vi "extract position data.vi"(0 "Receive data":string, 2 "Pre X_M":string, 3 "Pre Y_M":string, 4 "Pre Z_M":string, 5 "Pre X_A":string, 6 "Pre Y_A":string, 7 "Pre Z_A":string) -> (9 "X_A":string, 11 "Y_A":string, 14 "Address":string, 15 "Z_A":string, 16 "Function Code":string, 17 "A_A":string, 20 "X_M":string, 21 "Y_M":string, 23 "Z_M":string, 24 "A_M":string, 27 "CheckSumCorrect":bool)   [LabVIEW 2014, in "HPCNC.lvlib"]
uses:
  HPCNC.lvlib
  GetCncPosition.dll
  mosbusCheckSum.dll
panel:
  in  "dataToGet":i32
  out "length check":string
  out "ChkSumData":u32
  out "AaIdx":u8
  out "ZaIdx":u8
  out "YaIdx":u8
  out "XaIdx":u8
  out "AmIdx":u8
  out "ZmIdx":u8
  out "YmIdx":u8
  out "XmIdx":u8
  out "ChkSumCalculated":u8
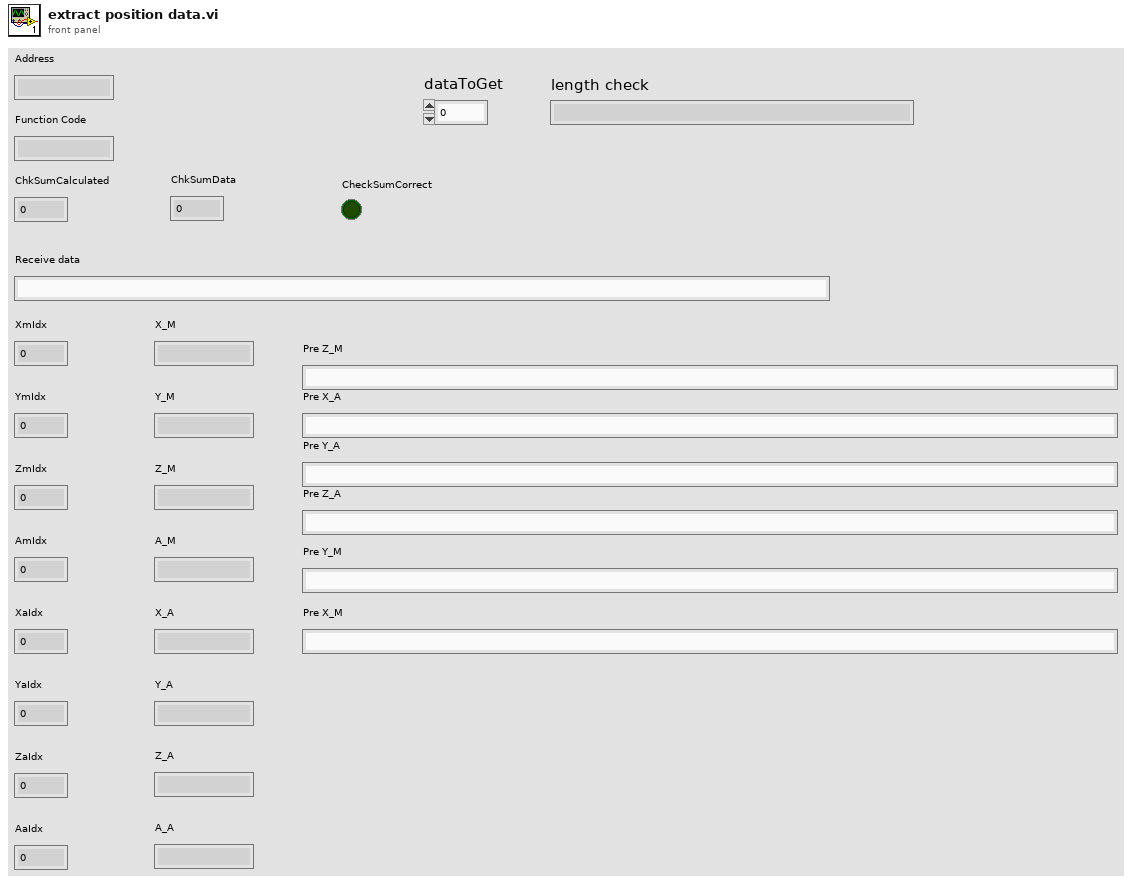
[diagram p1: front panel]
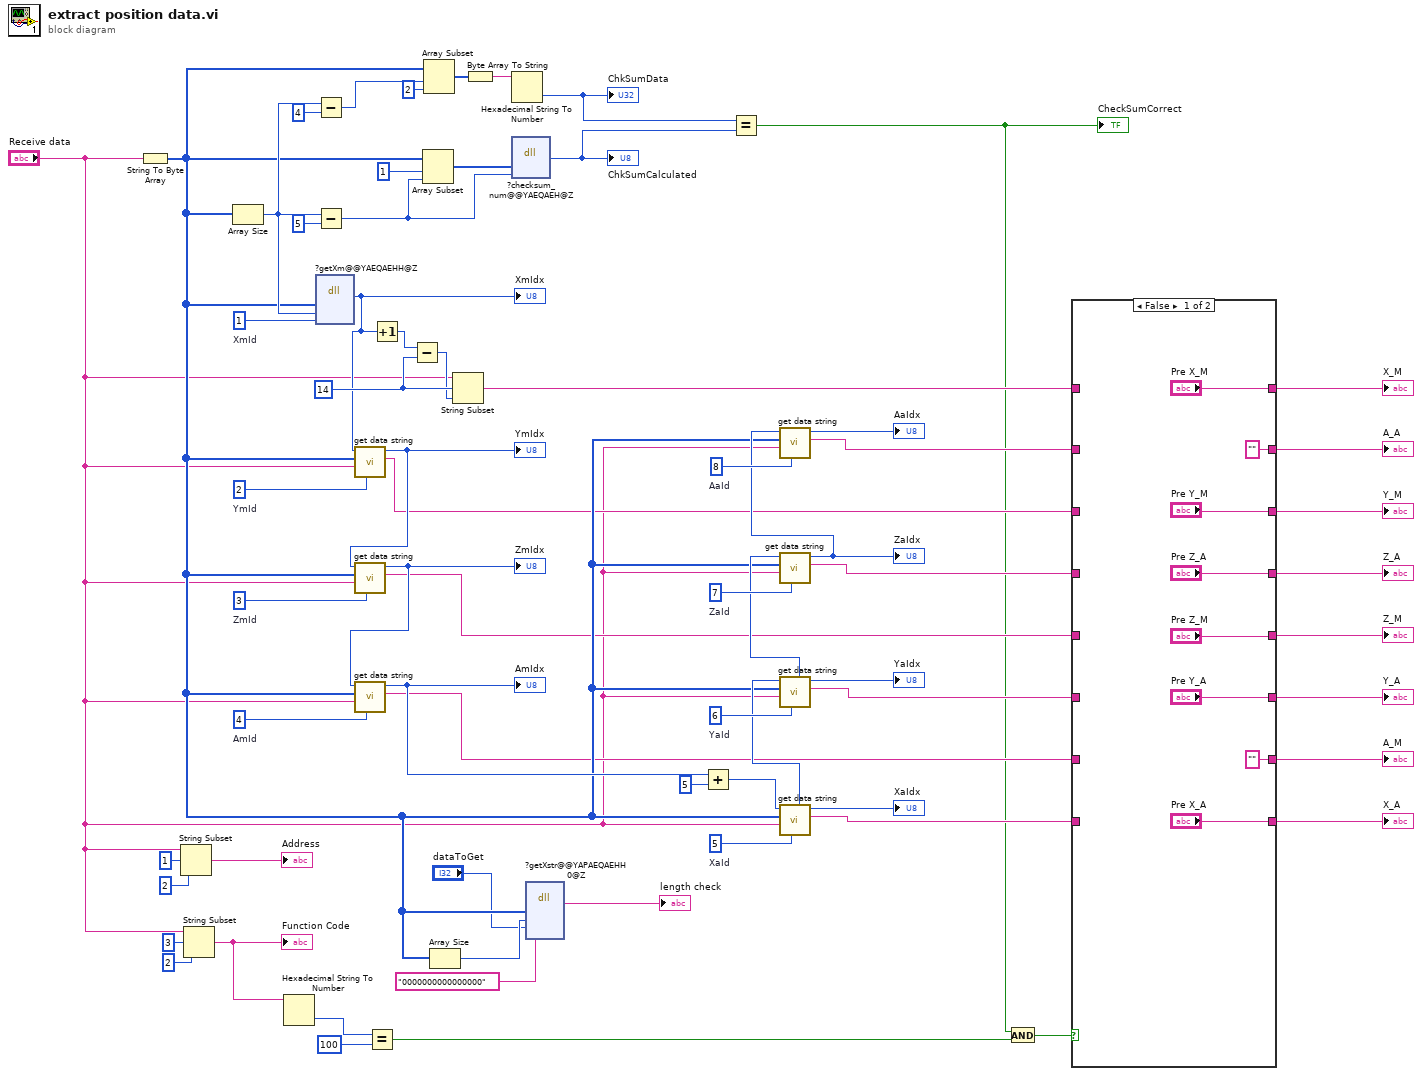
[diagram p0: block diagram]
diagram:
  w50 = 8  # AaId
  w51 = 7  # ZaId
  w52 = 6  # YaId
  w56 = 5  # XaId
  w58 = 4  # AmId
  w59 = 3  # ZmId
  w62 = 2  # YmId
  w63 = 1  # XmId
  w66 = 14 ("offset (0)")
  n1 = String To Byte Array(string="Receive data") -> (unsigned byte array=w28:u8[])
  n2 = String Subset(string="Receive data", offset (0)=1, length (rest)=2 ("length (rest)")) -> (substring=→"Address":string)
  n3 = String Subset(string="Receive data", offset (0)=3, length (rest)=2 ("length (rest)")) -> (substring=w23:string)
  "Function Code" <- w23
  n4 = Array Size(array=w28) -> (size(s)=w41:i32)
  n5 = Hexadecimal String To Number(string=w23) -> (number=w5:u32)  [unwired: 2 in, 1 out]
  n6 = Subtract(x=w41, y=4) -> (x-y=w39:i32)
  n7 = Subtract(x=w41, y=5) -> (x-y=w42:i32)
  n8 = dll-call lib="D:/Workspace/Giang/Labview/Minigantry With FS/SubVIs/GetCncPosition.dll" fn="?getXm@@YAEQAEHH@Z" label="dataindex"("arrayI"=w28, "size"=w41, "dataToGet"=w63) -> ("return type"=w61:u8)  [unwired: 6 in, 2 out]
  "XmIdx" <- w61
  n9 = call "get data string.vi"("dataToGet"=w62, "read buffer in"="Receive data", "unsigned byte array"=w28, "startIdx"=w61) -> ("read buffer out"=w16:string, "lastIdx"=w60:u8)  [unwired: 6 in]
  "YmIdx" <- w60
  n10 = call "get data string.vi"("dataToGet"=w59, "read buffer in"="Receive data", "unsigned byte array"=w28, "startIdx"=w60) -> ("read buffer out"=w12:string, "lastIdx"=w57:u8)  [unwired: 6 in]
  "ZmIdx" <- w57
  n11 = call "get data string.vi"("dataToGet"=w58, "read buffer in"="Receive data", "unsigned byte array"=w28, "startIdx"=w57) -> ("read buffer out"=w8:string, "lastIdx"=w54:u8)  [unwired: 6 in]
  "AmIdx" <- w54
  n12 = Equal?(x=w5, y=100) -> (x = y?=w2:bool)
  n13 = Increment(x=w61) -> (x+1=w64:u8)
  n14 = Subtract(x=w64, y=w66) -> (x-y=w65:i32)
  n15 = Array Subset(array=w28, index=1, length=w42) -> (w43:u8[])
  n16 = Array Subset(array=w28, index=w39, length=2) -> (w37:u8[])
  n17 = Array Size(array=w28) -> (size(s)=w27:i32)
  n18 = String Subset(string="Receive data", offset (0)=w66, length (rest)=w65) -> (substring=w20:string)
  n19 = Byte Array To String(unsigned byte array=w37) -> (string=w36:string)
  n20 = Hexadecimal String To Number(string=w36) -> (number=w35:u32)  [unwired: 2 in, 1 out]
  "ChkSumData" <- w35
  n21 = dll-call lib="D:/Workspace/Giang/Labview/Minigantry With FS/SubVIs/mosbusCheckSum.dll" fn="?checksum_num@@YAEQAEH@Z" label="ChkSum"("arrayI"=w43, "size"=w42) -> ("return type"=w34:u8)  [unwired: 5 in, 2 out]
  "ChkSumCalculated" <- w34
  n22 = dll-call lib="D:/Workspace/Giang/Labview/Minigantry With FS/SubVIs/GetCncPosition.dll" fn="?getXstr@@YAPAEQAEHH0@Z" label="Data index"("arrayI"=w28, "size"=w27, "dataToGet"="dataToGet", "returnArray"="0000000000000000") -> ("return type"=→"length check":string)  [unwired: 7 in, 2 out]
  n23 = Add(x=w54, y=u8 5) -> (x+y=w55:u8)
  n24 = Equal?(x=w35, y=w34) -> (x = y?=w3:bool)
  "CheckSumCorrect" <- w3
  n25 = call "get data string.vi"("dataToGet"=w56, "read buffer in"="Receive data", "unsigned byte array"=w28, "startIdx"=w55) -> ("read buffer out"=w6:string, "lastIdx"=w46:u8)  [unwired: 6 in]
  "XaIdx" <- w46
  n26 = call "get data string.vi"("dataToGet"=w52, "read buffer in"="Receive data", "unsigned byte array"=w28, "startIdx"=w46) -> ("read buffer out"=w10:string, "lastIdx"=w47:u8)  [unwired: 6 in]
  "YaIdx" <- w47
  n27 = call "get data string.vi"("dataToGet"=w51, "read buffer in"="Receive data", "unsigned byte array"=w28, "startIdx"=w47) -> ("read buffer out"=w14:string, "lastIdx"=w48:u8)  [unwired: 6 in]
  "ZaIdx" <- w48
  n28 = call "get data string.vi"("dataToGet"=w50, "read buffer in"="Receive data", "unsigned byte array"=w28, "startIdx"=w48) -> ("read buffer out"=w18:string, "lastIdx"=→"AaIdx":u8)  [unwired: 6 in]
  n29 = And(x=w3, y=w2) -> (x .and. y?=w1:bool)
  n30 = case shown="False" w1 {
    tunnel: ["Pre X_M" w82] -> w21
    tunnel: w20 -> [_ w82]
    tunnel: ["" ("read buffer out") w81] -> w19
    tunnel: w18 -> [_ w81]
    tunnel: ["Pre Y_M" w80] -> w17
    tunnel: w16 -> [_ w80]
    tunnel: ["Pre Z_A" w79] -> w15
    tunnel: w14 -> [_ w79]
    tunnel: ["Pre Z_M" w78] -> w13
    tunnel: w12 -> [_ w78]
    tunnel: ["Pre Y_A" w77] -> w11
    tunnel: w10 -> [_ w77]
    tunnel: ["" ("read buffer out") w76] -> w9
    tunnel: w8 -> [_ w76]
    tunnel: ["Pre X_A" w75] -> w7
    tunnel: w6 -> [_ w75]
    frame False {
    }
    frame True {
    }
  }
  "X_M" <- w21
  "Y_M" <- w17
  "Z_M" <- w13
  "A_M" <- w9
  "X_A" <- w7
  "Y_A" <- w11
  "Z_A" <- w15
  "A_A" <- w19
